vi "Transport Teardown.vi"(9 "Address":refnum<event-registration>, 10 "Transport":refnum<user-event>) -> (2 "Unheard Msgs":refnum<class "Msg.lvclass">[](array[class]))   [LabVIEW 2020, in "jettl.lvlib"]
uses:
  jettl.lvlib
  Msg/Msg.lvclass
  Relation.ctl
  Teller.ctl
  Msg Input/Msg Input.lvclass
  Msg Output/Msg Output.lvclass
  Msg Attributes.ctl
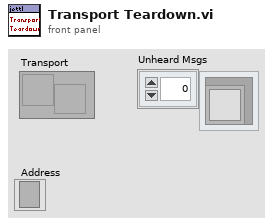
[diagram p1: front panel]
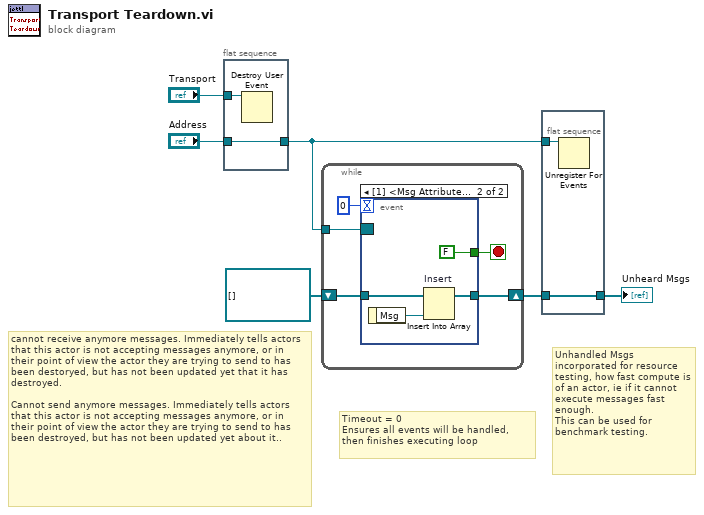
[diagram p0: block diagram]
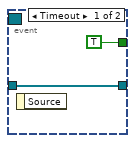
[diagram p2: hidden frame]
diagram:
  # "Unhandled Msgs incorporated for resource testing, how fast compute is of an actor, ie if it cannot execute messages fast enough.\nThis can be used for benchmark testing."
  # "Timeout = 0\nEnsures all events will be handled, then finishes executing loop"
  # "cannot receive anymore messages. Immediately tells actors that this actor is not accepting messages anymore, or in their point of view the actor they are trying to send to has been destoryed, but has not been updated yet that it has destroyed.\n\nCannot send anymore messages. Immediately tells actors that this actor is not accepting messages anymore, or in their point of view the actor they are trying to send to has been destroyed, but has not been updated yet about it.."
  n1 = flat-sequence {
    tunnel: [w8] -> w2
    tunnel: "Address" -> [w8]
    tunnel: "Transport" -> [w7]
    frame #0 {
      n2 = Destroy User Event(user event=w7) -> ()  [unwired: 1 in, 1 out]
    }
  }
  n3 = while {
    shift-right: [w12] -> w4
    shift-left: refnum<class "Msg.lvclass">[] [] -> [w13]
    tunnel: w2 -> [w11]
    stop <- w10 stop-if-true
    n4 = event shown="[1] <Msg Attributes>: User Event" {
      selector: w11 -> [_ _]
      dyn-events: _ -> [_ _]
      timeout: 0 -> [_ _]
      tunnel: w13 -> [w15 w19]
      tunnel: [w15 w18] -> w12
      tunnel: [TRUE FALSE] -> w10
      event Timeout {
        n5 = event-data() -> ()  [unwired: 1 in, 1 out]
      }
      event User Event {
        n6 = event-data() -> ("Msg"=w16:refnum<class "Msg.lvclass">)  [unwired: 1 in]
        n7 = Insert Into Array "Insert"(array=w19, new element=w16) -> (w18:refnum<class "Msg.lvclass">[])  [unwired: 1 in]
      }
    }
  }
  n8 = flat-sequence {
    tunnel: w2 -> [w21]
    tunnel: [w20] -> w5
    tunnel: w4 -> [w20]
    frame #0 {
      n9 = Unregister For Events(event registration refnum=w21) -> ()  [unwired: 1 in, 1 out]
    }
  }
  "Unheard Msgs" <- w5
